vi "DeviceIsOpen.vi"(6 "Delay between send and receive [ms]":i32=100, 8 "error in (no error)":errorcluster, 11 "CCD in":refnum<class "CCD.lvclass">) -> (0 "error out":errorcluster, 1 "ID":i32, 2 "device is open?":bool, 3 "CCD out":refnum<class "CCD.lvclass">)   [LabVIEW 2023, in "CCD.lvclass"]
uses:
  CCD.lvclass
  GenericDevice/GenericDevice.lvclass
  CCD.lvclass/CCD.ctl
panel:
  # "Connector Pane"
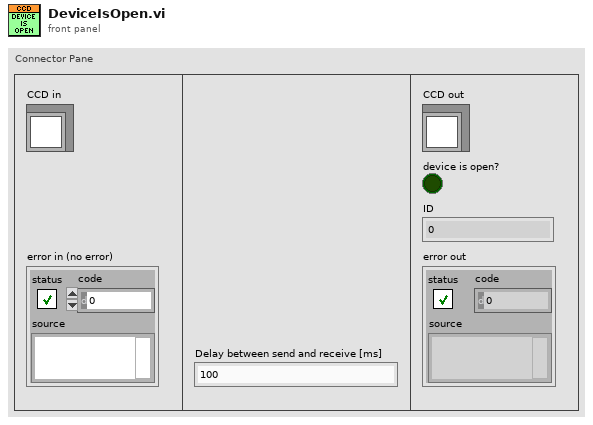
[diagram p1: front panel]
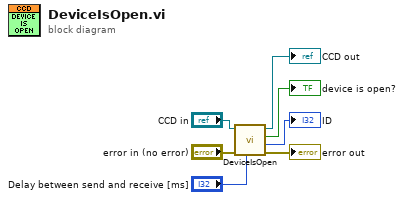
[diagram p0: block diagram]
diagram:
  n1 = call-parent "DeviceIsOpen.vi"("Delay between send and receive [ms]"="Delay between send and receive [ms]", "error in (no error)"="error in (no error)", "GenericDevice in"="CCD in") -> ("error out"=→"error out":errorcluster, "ID"=→"ID":i32, "device is open?"=→"device is open?":bool, "GenericDevice out"=→"CCD out":refnum<class "CCD.lvclass">)  [unwired: 5 in]
